vi "BRig_FPGA_resetOutputs_PortC.vi"   [LabVIEW 2014]
uses:
  <vilib>/rvi/eio/common/nirviEmuTemplateMethod_errors.vi
  <vilib>/eio/EIONode/EIONode.xnode
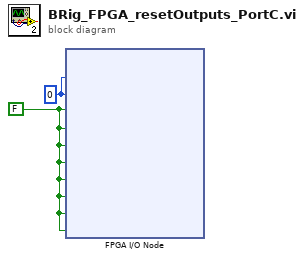
[diagram p0: block diagram]
diagram:
  w1 = i16 0 ("ConnectorA/AO0")
  w2 = FALSE ("ConnectorA/DIO3")
  n1 = xnode "FPGA I/O Node"("ConnectorC/AO0"=w1, "ConnectorC/AO1"=w1, "ConnectorC/DIO0"=w2, "ConnectorC/DIO1"=w2, "ConnectorC/DIO2"=w2, "ConnectorC/DIO3"=w2, "ConnectorC/DIO4"=w2, "ConnectorC/DIO5"=w2, "ConnectorC/DIO6"=w2, "ConnectorC/DIO7"=w2) -> ()  [unwired: 10 in, 10 out]
